vi "CAP Forward Masking.vi"(11 "State":T7={"Experimenter"="XYZ", "Number"=999, "Right"="Right", "Left"="Left", "Data Folder"=path "C:/Data/XYZ DATA/XYZ999", "State File"=path "C:/Data/XYZ DATA/XYZ999/Experiment State.txt", "Version Info"="CFTS VIs: V1.2 (Rev. 132)\nExperiment VIs: 132\nLabVIEW.exe V10.0 (2010)\nDAQmx V9.1", "End Exposure Time"=-1.0, "Exposure Duration"="", "Run #"={"CAP"=0, "ABR"=0, "DP"=0, "VsEP"=0, "MeasSeq"=0, "SubSeq"=0, "SFOAE"=0}}) -> (3 "State Out":T7={"Experimenter"="XYZ", "Number"=999, "Right"="Right", "Left"="Left", "Data Folder"=path "C:/Data/XYZ DATA/XYZ999", "State File"=path "C:/Data/XYZ DATA/XYZ999/Experiment State.txt", "Version Info"="CFTS VIs: V1.2 (Rev. 132)\nExperiment VIs: 132\nLabVIEW.exe V10.0 (2010)\nDAQmx V9.1", "End Exposure Time"=-1.0, "Exposure Duration"="", "Run #"={"CAP"=0, "ABR"=0, "DP"=0, "VsEP"=0, "MeasSeq"=0, "SubSeq"=0, "SFOAE"=0}})   [LabVIEW 2020]
uses:
  CFTS Main Panel SubVIs/CFTS-Experiment State.ctl
  epl-vi-lib/Utility VIs/Type Defs/Left-Right ring.ctl
  Typedefs/CAPFM-Control References.ctl
  Typedefs/CAPFM-All Params.ctl
  Typedefs/CAPFM-Probe Params.ctl
  Typedefs/CAPFM-Masker Params.ctl
  Typedefs/CAPFM-Seq Params.ctl
  Typedefs/CAPFM-Timing Params.ctl
  Typedefs/CAPFM-Response Params.ctl
panel:
  out "Pause Msg":string
  in  "Pause":bool
  out "Attempted":i32
  in  "OverRide":bool
  in  "Threshold (uV)":dbl=15.0
  out "Reject":bool
  out "Decr":cluster{"Interval":dbl[], "Decrement":dbl[]}(graph)
  out "Refs":T1
  out "Mags":cluster{dbl[], dbl[]}[](graph)
  out "CAP":cluster{i32, "dx":dbl, "Array":dbl[][]}(graph)
  in  "Notes":string
  in  "Response":T2={"Gain"=10000.0, "Fs (Hz)"=0.0, "Save traces?"=FALSE, "Window (ms)"=8.0, "Filter?"=FALSE}
  out "Acquired":i32
  out "Interval (ms)":dbl
  in  "Timing":T3={"Rep rate (Hz)"=0.0, "TRecover (ms)"=200.0, "Method"=0} {"Method" items=["Recovery (ms)", "Rep rate (/s)"]}
  in  "Probe":T4={"Freq (kHz)"=10.0, "dB SPL"=50.0, "AltPol"=TRUE, "Dur (ms)"=5.0}
  in  "Sequence":cluster{"Intervals (ms)":string, "NAvgs":i32}={"Intervals (ms)"="2;4;8;16;32;64;128;256;512", "NAvgs"=10}
  in  "Ear":T5
  in  "Masker":T6={"dB SPL"=50.0, "Dur (ms)"=100.0, "InvFilt"=FALSE}
  out "User":string="XYZ"
  out "Run #":u16
  out "ID #":u16=999
  out "running":bool
  in  "Exit":bool
  in  "Go":bool
  out "exit signal":bool
  out "Abort":bool
  in  "Stop":bool
  # "Probe"
  # "Masker"
  # "Intervals"
  # "Response"
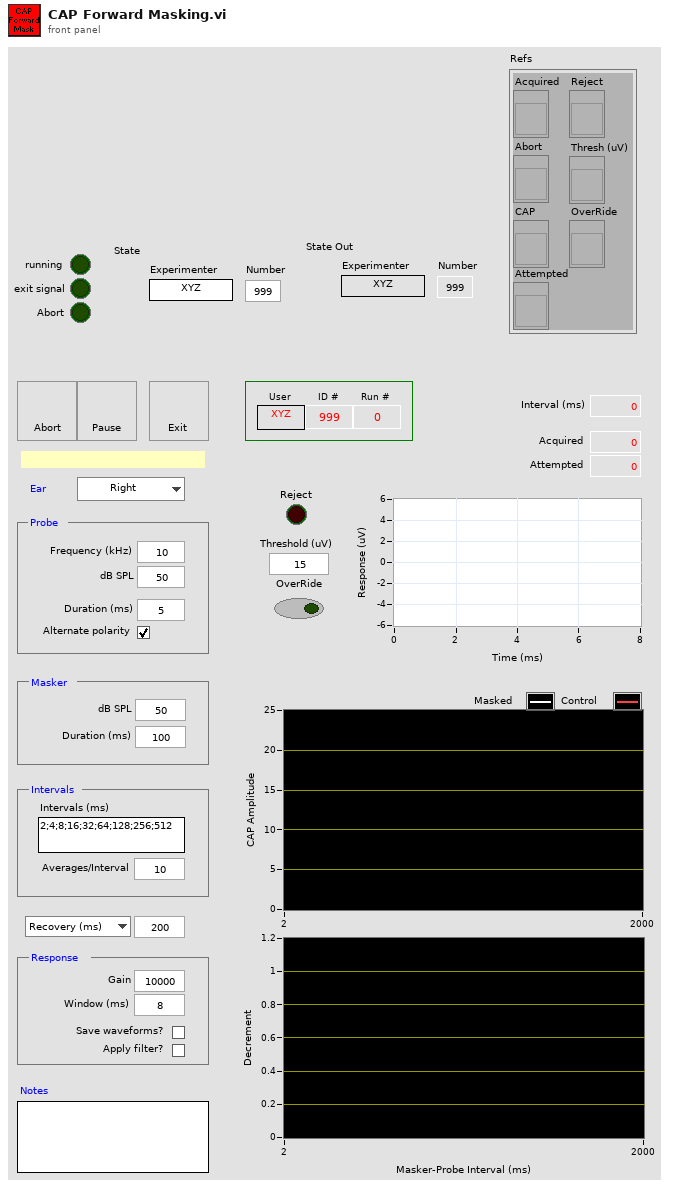
[diagram p1: front panel]
types:
  T1 = typedef "CAPFM-Control References.ctl" = cluster{"Acquired":refnum<vi>, "Abort":refnum<vi>, "CAP":refnum<vi>, "Reject":refnum<vi>, "Thresh (uV)":refnum<vi>, "OverRide":refnum<vi>, "Attempted":refnum<vi>}
  T2 = cluster{"Gain":dbl, "Fs (Hz)":dbl, "Save traces?":bool, "Window (ms)":dbl, "Filter?":bool}
  T3 = cluster{"Rep rate (Hz)":dbl, "TRecover (ms)":dbl, "Method":u16}
  T4 = cluster{"Freq (kHz)":dbl, "dB SPL":dbl, "AltPol":bool, "Dur (ms)":dbl}
  T5 = typedef "Left-Right ring.ctl" = enum16{"Right", "Left"}
  T6 = cluster{"dB SPL":dbl, "Dur (ms)":dbl, "InvFilt":bool}
  T7 = typedef "CFTS-Experiment State.ctl" = cluster{"Experimenter":string, "Number":u32, "Right":string, "Left":string, "Data Folder":path, "State File":path, "Version Info":string, "End Exposure Time":dbl, "Exposure Duration":string, "Run #":cluster{"CAP":i16, "ABR":i16, "DP":i16, "VsEP":i16, "MeasSeq":i16, "SubSeq":i16, "SFOAE":i16}}
  T8 = typedef "CAPFM-All Params.ctl" = cluster{"Ear":T5, "Probe":T9, "Masker":T10, "Sequence":T11, "Fs (Hz)":dbl, "Timing":T12, "Response":T13}
  T9 = typedef "CAPFM-Probe Params.ctl" = cluster{"Freq (kHz)":dbl, "dB SPL":dbl, "AltPol":bool, "Dur (ms)":dbl}
  T10 = typedef "CAPFM-Masker Params.ctl" = cluster{"dB SPL":dbl, "Dur (ms)":dbl, "InvFilt":bool}
  T11 = typedef "CAPFM-Seq Params.ctl" = cluster{"List (ms)":string, "NAvgs":i32}
  T12 = typedef "CAPFM-Timing Params.ctl" = cluster{"Rep rate (Hz)":dbl, "TRecover (ms)":dbl, "Method":enum16{"Fixed recovery", "Fixed rep rate"}}
  T13 = typedef "CAPFM-Response Params.ctl" = cluster{"Gain":dbl, "Fs (Hz)":dbl, "Save traces?":bool, "Window (ms)":dbl, "Filter?":bool}
  T14 = typedef "CAPFM-Runtime Data.ctl" = cluster{"Offset":i32, "AI Npts":i32, "Gain":dbl, "WinPts":i32, "NAvg":i32, "dt (ms)":dbl, "FiltCoef":dbl[]}
  T15 = typedef "Stimulus Channel (Full).xctl/Full Stimulus Channel Data.ctl" = cluster{"Waveform":T16, "Filter":T33, "Burst":T35, "Level":T36, "Name":string, "Advanced":T38, "SAM":T39}
  T16 = typedef "Waveform XCtl.xctl/Waveform Data.ctl" = cluster{"Type":T17, "Tone":T18, "Pulse Train":T19, "Noise":T22, "File":T23, "FMSweep":T24, "Chirp Train":T25, "Complex Tone":cluster{"Params":T27, "Data":T29}, "Moving Ripple":T30}
  T17 = typedef "Waveform Enum.ctl" = enum16{"OFF", "Tone", "Noise", "Pulse Train", "File", "FM Sweep", "Chirp Train", "Complex Tone", "FM Tone", "Moving Ripple"}
  T18 = typedef "Tone Params.ctl" = cluster{"Frequency (kHz)":dbl, "Last Freq":dbl, "Last Phase":dbl}
  T19 = typedef "Pulse Train Params.ctl" = cluster{"Pulse width (us)":dbl, "Pulse rate (Hz)":dbl, "Gap (ms)":dbl, "Polarity":T20, "PT State":T21, "Asynch":bool}
  T20 = typedef "Pulse Polarity.ctl" = enum16{"POS", "NEG", "POS-NEG", "NEG-POS"}
  T21 = typedef "PT-Continuous State.ctl" = cluster{"Template":dbl[], "Nperiod":i32, "Index":i32, "Pulse Rate (Hz)":dbl, "Phase (cycles)":dbl, "Noff":i32}
  T22 = typedef "Noise Params.ctl" = cluster{"InvFilt":bool, "Noise":dbl[], "CurPt":i32, "Aweight":bool, "Seed":i32, "afile":path}
  T23 = typedef "StimFile-Params.ctl" = cluster{"Filename":path, "Signal":dbl[], "Channel":i32, "stream":bool, "offset":i32, "nreps":i32, "loops":i32, "Randomize":bool, "order":i32[], "Seed":i32, "Tokens":i32}
  T24 = typedef "FM Sweep Params.ctl" = cluster{"Rate (oct/s)":dbl, "Fmin (Hz)":dbl, "Fmax (Hz)":dbl, "Ramp (ms)":dbl, "Linear":bool}
  T25 = typedef "Chirp Train.ctl" = cluster{"Params":T26, "Data":cluster{"WF":dbl[]}}
  T26 = typedef "Chirp Train Params.ctl" = cluster{"Fmin (kHz)":dbl, "Fmax (kHz)":dbl, "Compensate":bool, "Duration (ms)":dbl}
  T27 = typedef "CT-Params.ctl" = cluster{"F0 (Hz)":dbl, "Band":cluster{"Flow (Hz)":dbl, "Fhigh (Hz)":dbl}, "Phase":T28, "Min F0 (Hz)":dbl, "Max F0 (Hz)":dbl, "ContinRandPhase":bool, "Max peak factor":dbl, "Max mod depth":dbl, "MinHarmNum":i32, "MaxHarmNum":i32, "Level Mode":enum16{"per component", "overall rms"}, "% jitter":dbl}
  T28 = typedef "CT-Phase Enum.ctl" = enum16{"Cosine", "Random", "Alternating"}
  T29 = typedef "CT-Runtime Data.ctl" = cluster{"Ncomp":i32, "MinHarm":i32, "Phase":dbl[], "Amplitude":dbl[], "Npts/frame":i32, "Last F0":dbl, "Fmin":dbl, "Fmax":dbl, "Lslope":dbl, "randphase":bool, "overall rms":bool, "fmult":dbl[], "jittered":bool}
  T30 = typedef "Moving Ripple.ctl" = cluster{"Params":T31, "Data":T32}
  T31 = typedef "Moving Ripple.Params.ctl" = cluster{"Fmin":dbl, "Fmax":dbl, "Density":dbl, "Velocity":dbl, "Depth":dbl, "Phase":dbl, "Comp/oct":i32}
  T32 = typedef "Moving Ripple.Data.ctl" = cluster{"Freq":dbl[], "A":dbl[], "phase":dbl[], "Phase":dbl}
  T33 = typedef "Advanced Filter XCtl.xctl/Filter Data.ctl" = cluster{"Type":enum16{"Lowpass", "Highpass", "Bandpass", "Bandstop", "OFF"}, "CF (kHz)":dbl, "BW (kHz)":dbl, "Cascade":bool, "Quadrature":bool, "Scale Factor":dbl, "Stages":cluster{"IIR Filter":cluster{"filter structure":enum32{"IIR 2nd Order", "IIR 4th Order"}, "Reverse Coefficients":dbl[], "Forward Coefficients":dbl[]}, "State":dbl[]}[], "Class":enum16{"Elliptic", "Butterworth"}, "Order":i32, "BWUnits":T34}
  T34 = typedef "Filter-Bandwidth Units.ctl" = enum16{"Linear", "Octaves", "Min-Max"}
  T35 = typedef "Burst Control.xctl/Burst Data.ctl" = cluster{"Active":bool, "Delay (ms)":dbl, "Duration (ms)":dbl, "Ramp (ms)":dbl, "Rate (Hz)":dbl, "Trepeat (ms)":dbl, "Repeat":bool}
  T36 = typedef "Level XCtl.xctl/Level Data.ctl" = cluster{"Level":dbl, "Units":T37, "Max":dbl, "Multiplier":dbl, "Cal File":path, "Cal":cluster{"Freq (Hz)":dbl[], "Mag (dB SPL)":dbl[], "Phase (deg)":dbl[]}}
  T37 = typedef "Level Units.ctl" = enum16{"dB atten", "dB SPL", "dB re 1 Vrms", "dB V/Hz½", "mW", "dB HL", "Volts", "dB mW"}
  T38 = typedef "Advanced Stimulus Options.xctl/Advanced Stimulus Options.ctl" = cluster{"Rep Mask":string, "AltPol":bool, "Var":string, "Expr":string, "Persist":bool}
  T39 = typedef "SAM Params.ctl" = cluster{"Active":bool, "Frequency (Hz)":dbl, "Depth":dbl, "Init Phase (cycles)":dbl, "phase (degrees)":dbl, "Asynch":bool}
  T40 = typedef "CAPFM-Analysis State.ctl" = cluster{"CAPs":dbl[][], "Interval":dbl[], "Control":dbl[], "Masked":dbl[], "Decrement":dbl[], "Order":i32[]}
  T41 = cluster{"Acquired":refnum<vi>, "Abort":refnum<vi>, "CAP":refnum<vi>, "Reject":refnum<vi>, "Threshold (uV)":refnum<vi>, "OverRide":refnum<vi>, "Attempted":refnum<vi>}
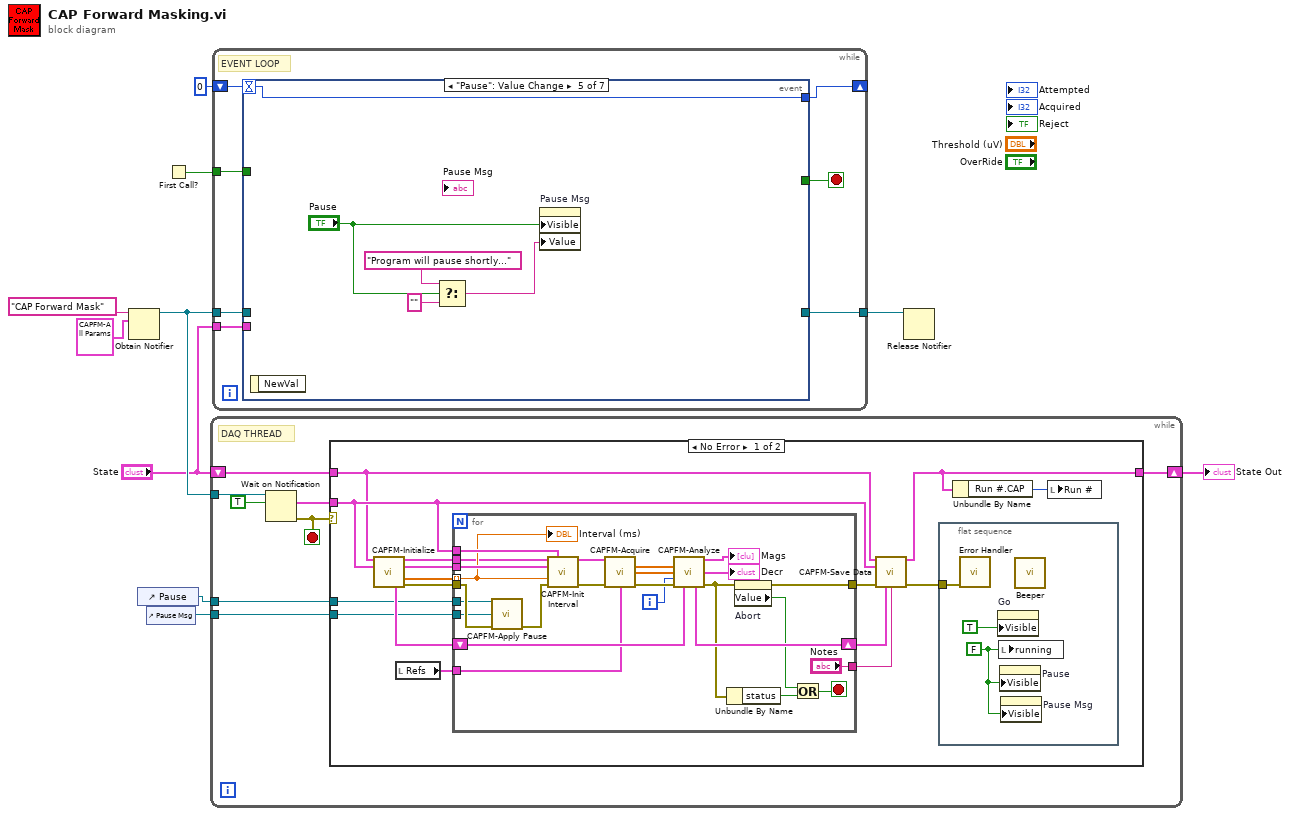
[diagram p0: block diagram]
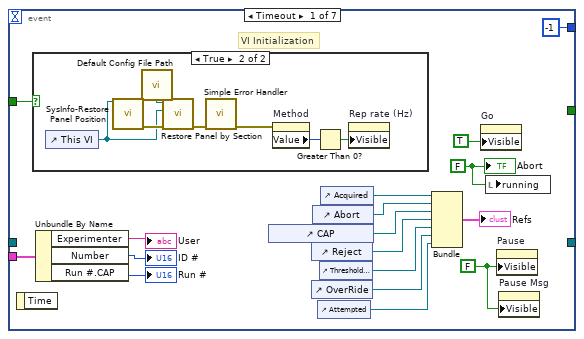
[diagram p3: hidden frame]
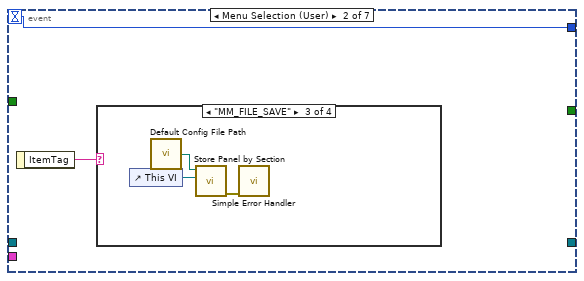
[diagram p5: hidden frame]
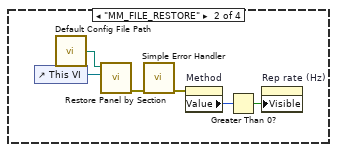
[diagram p7: hidden frame]
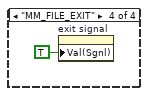
[diagram p8: hidden frame]
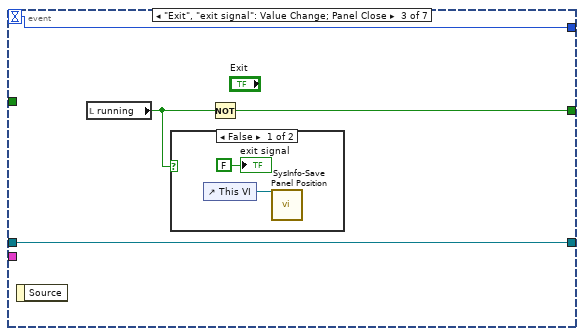
[diagram p9: hidden frame]
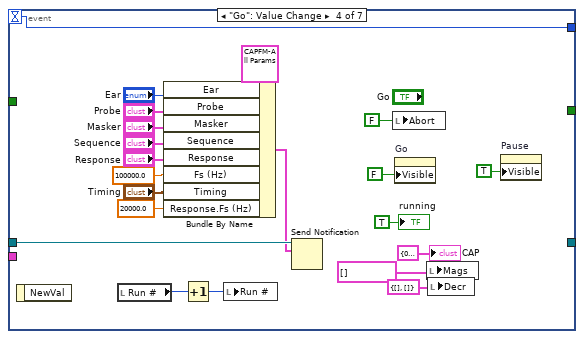
[diagram p11: hidden frame]
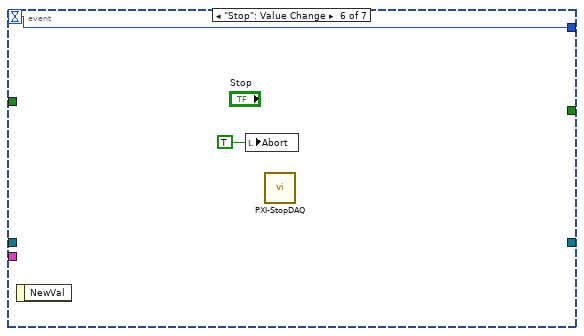
[diagram p12: hidden frame]
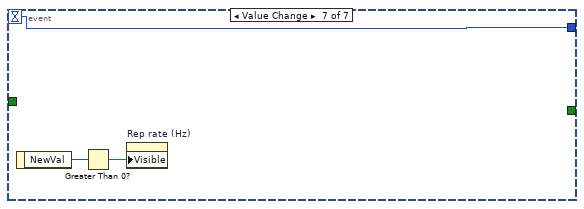
[diagram p13: hidden frame]
diagram:
  n1 = Obtain Notifier(name (unnamed)="CAP Forward Mask", notification data type=T8 {"Ear"=enum."Right", "Probe"={"Freq (kHz)"=0.0, "dB SPL"=0.0, "AltPol"=FALSE, "Dur (ms)"=0.0}, "Masker"={"dB SPL"=0.0, "Dur (ms)"=0.0, "InvFilt"=FALSE}, "Sequence"={"List (ms)"="", "NAvgs"=0}, "Fs (Hz)"=0.0, "Timing"={"Rep rate (Hz)"=0.0, "TRecover (ms)"=0.0, "Method"=enum."Fixed recovery"}, "Response"={"Gain"=0.0, "Fs (Hz)"=0.0, "Save traces?"=FALSE, "Window (ms)"=0.0, "Filter?"=FALSE}} ("CAPFM Params")) -> (notifier out=w6:refnum<notifier>)  [unwired: 2 in, 2 out]
  n2 = control-ref of="Pause"() -> (w2:refnum<vi>)
  n3 = control-ref of="Pause Msg"() -> (w1:refnum<vi>)
  n4 = First Call?() -> (First Call?: T/F=w7:bool)
  n5 = while {
    tunnel: w6 -> [w17]
    shift-right: [w13] -> w3
    shift-left: "State" -> [w14]
    tunnel: w2 -> [w12]
    tunnel: w1 -> [w11]
    stop <- w15 stop-if-true
    # "DAQ THREAD"
    n6 = Wait on Notification(notifier=w17, ignore previous (F)=TRUE) -> (notification=w16:T8, error out=w15:errorcluster)  [unwired: 2 in, 2 out]
    n7 = case shown="No Error" w15 {
      tunnel: w16 -> [w27 _]
      tunnel: w14 -> [w26 w63]
      tunnel: [w25 w63] -> w13
      tunnel: w12 -> [w20 _]
      tunnel: w11 -> [w19 _]
      frame No Error {
        n8 = call "CAPFM-Initialize.vi"("Expt State"=w26, "CAPFM Params"=w27) -> ("Runtime"=w21:T14, "StimChans"=w31:T15[], "Intervals (ms)"=w34:dbl[], "Analysis"=w33:T40, "error out"=w32:errorcluster)  [unwired: 9 in]
        n9 = local read "Refs"() -> (w22:T1)
        n10 = for {
          tunnel: w34 -> [w40] mode=indexing
          shift-right: [w55] -> w29
          shift-left: w33 -> [w56]
          tunnel: w32 -> [w37]
          tunnel: w31 -> [w59]
          tunnel: w27 -> [w41]
          tunnel: [w43] -> w30
          tunnel: ["Notes"] -> w28
          tunnel: w22 -> [w50]
          tunnel: w21 -> [w39]
          tunnel: w20 -> [w36]
          tunnel: w19 -> [w35]
          i -> [w49]
          stop <- w46 stop-if-true
          n11 = call "CAPFM-Apply Pause.vi"("Pause Ref"=w36, "Pause Msg Ref"=w35, "error in (no error)"=w37) -> ("error out"=w38:errorcluster)  [unwired: 12 in]
          n12 = call "CAPFM-Init Interval.vi"("Runtime In"=w39, "CAPFM Params"=w41, "StimChans"=w59, "Interval (ms)"=w40, "error in (no error)"=w38) -> ("Runtime Out"=w54:T14, "error out"=w58:errorcluster)  [unwired: 9 in]
          n13 = call "CAPFM-Acquire.vi"("Runtime"=w54, "error in (no error)"=w58, "Refs"=w50) -> ("Control"=w53:dbl[], "Masked"=w52:dbl[], "error out"=w57:errorcluster)  [unwired: 10 in]
          n14 = call "CAPFM-Analyze.vi"("Control"=w53, "Masked"=w52, "Index"=w49, "error in (no error)"=w57, "Analysis"=w56) -> ("Mags"=→"Mags":cluster{"Interval":dbl[], "Control":dbl[]}[], "Decrement"=→"Decr":cluster{"Interval":dbl[], "Decrement":dbl[]}, "Analysis Out"=w55:T40, "error out"=w47:errorcluster)  [unwired: 7 in]
          n15 = Unbundle By Name(w47) -> ("status"=w45:bool)
          n16 = property on="Abort" class="Bool (strict)"(error in=w47) -> (error out=w43:errorcluster, "Value"=w42:bool)  [unwired: 1 in, 1 out]
          n17 = Or(x=w42, y=w45) -> (x .or. y?=w46:bool)
          "Interval (ms)" <- w40
        }
        n18 = call "CAPFM-Save Data.vi"("Expt State"=w26, "CAPFM Params"=w27, "error in"=w30, "Analysis"=w29, "Notes"=w28) -> ("Expt State Out"=w25:T7, "error out"=w23:errorcluster)  [unwired: 9 in]
        n19 = flat-sequence {
          tunnel: w23 -> [w61]
          frame #0 {
            w60 = FALSE ("running")
            n20 = call "Error Handler.vi"("error in (no error)"=w61) -> ()  [unwired: 13 in, 2 out]
            n21 = property on="Go" class="Bool"("Visible"=TRUE) -> ()  [unwired: 2 in, 2 out]
            n22 = local write "running"(w60) -> ()
            n23 = property on="Pause" class="Bool (strict)"("Visible"=w60) -> ()  [unwired: 2 in, 2 out]
            n24 = property on="Pause Msg" class="Str"("Visible"=w60) -> ()  [unwired: 2 in, 2 out]
            n25 = call "Beeper.vi"() -> ()  [unwired: 5 in, 1 out]
          }
        }
        n26 = Unbundle By Name(w25) -> ("Run #.CAP"=w24:i16)
        n27 = local write "Run #"(w24) -> ()
      }
      frame Error {
      }
    }
  }
  "State Out" <- w3
  n28 = while {
    tunnel: w6 -> [w70]
    tunnel: [w68] -> w10
    shift-right: [w66] -> _
    shift-left: 0 -> [w67]
    tunnel: w7 -> [w65]
    tunnel: "State" -> [w64]
    stop <- w69 stop-if-true
    # "EVENT LOOP"
    n29 = event shown="[4] \"Pause\": Value Change" {
      selector: _ -> [_ _ _ _ _ _ _]
      dyn-events: _ -> [_ _ _ _ _ _ _]
      timeout: w67 -> [_ w95 w109 w131 w138 w139 w143]
      tunnel: w70 -> [_ _ w110 w133 _ _ _]
      tunnel: [_ _ w107 _ _ _ _] -> w69
      tunnel: [_ _ w110 _ _ _ _] -> w68
      tunnel: [-1 w95 w109 w131 w138 w139 w143] -> w66
      tunnel: w65 -> [w84 _ _ _ _ _ _]
      tunnel: w64 -> [w83 _ _ _ _ _ _]
      event Timeout {
        w71 = FALSE ("Visible")
        w85 = FALSE ("Abort")
        # "VI Initialization"
        n30 = event-data() -> ()  [unwired: 1 in, 1 out]
        n31 = case shown="True" w84 {
          frame False {
          }
          frame True {
            n32 = control-ref of="This VI"() -> (w88:refnum<vi>)
            n33 = call "SysInfo-Restore Panel Position.vi"("VI Refnum"=w88) -> ("error out"=w92:errorcluster)  [unwired: 12 in, 2 out]
            n34 = call "Default Config File Path.vi"() -> ("Default config file name"=w93:path)
            n35 = call "Restore Panel by Section.vi"("error in (no error)"=w92, "VI reference"=w88, "Path (dialog)"=w93) -> ("Error Out"=w94:errorcluster)  [unwired: 8 in]
            n36 = call <vilib>:"Simple Error Handler.vi"("error in (no error)"=w94) -> ("error out"=w91:errorcluster)  [unwired: 4 in, 4 out]
            n37 = property on="Method" class="Ring (strict)"(error in=w91) -> ("Value"=w89:u16)  [unwired: 1 in, 2 out]
            n38 = Greater Than 0?(x=w89) -> (x > 0?=w90:bool)
            n39 = property on="Rep rate (Hz)" class="DigNum (strict)"("Visible"=w90) -> ()  [unwired: 2 in, 2 out]
          }
        }
        n40 = Unbundle By Name(w83) -> ("Experimenter"=→"User":string, "Number"=→"ID #":u32, "Run #.CAP"=→"Run #":i16)
        n41 = control-ref of="CAP"() -> (w77:refnum<vi>)
        n42 = control-ref of="Reject"() -> (w74:refnum<vi>)
        n43 = control-ref of="OverRide"() -> (w76:refnum<vi>)
        n44 = control-ref of="Abort"() -> (w78:refnum<vi>)
        n45 = control-ref of="Attempted"() -> (w73:refnum<vi>)
        n46 = control-ref of="Threshold (uV)"() -> (w75:refnum<vi>)
        n47 = control-ref of="Acquired"() -> (w79:refnum<vi>)
        n48 = Bundle("Acquired"=w79, "Abort"=w78, "CAP"=w77, "Reject"=w74, "Threshold (uV)"=w75, "OverRide"=w76, "Attempted"=w73) -> (→"Refs":T41)  [unwired: 1 in]
        n49 = property on="Go" class="Bool"("Visible"=TRUE) -> ()  [unwired: 2 in, 2 out]
        n50 = local write "running"(w85) -> ()
        n51 = property on="Pause" class="Bool (strict)"("Visible"=w71) -> ()  [unwired: 2 in, 2 out]
        n52 = property on="Pause Msg" class="Str"("Visible"=w71) -> ()  [unwired: 2 in, 2 out]
        "Abort" <- w85
      }
      event Menu Selection (User) {
        n53 = event-data() -> ("ItemTag"=w96:string)  [unwired: 1 in]
        n54 = case shown="\"MM_FILE_SAVE\"" w96 {
          frame "False", Default {
          }
          frame "MM_FILE_RESTORE" {
            n55 = control-ref of="This VI"() -> (w101:refnum<vi>)
            n56 = call "Default Config File Path.vi"() -> ("Default config file name"=w100:path)
            n57 = call "Restore Panel by Section.vi"("VI reference"=w101, "Path (dialog)"=w100) -> ("Error Out"=w102:errorcluster)  [unwired: 9 in]
            n58 = call <vilib>:"Simple Error Handler.vi"("error in (no error)"=w102) -> ("error out"=w97:errorcluster)  [unwired: 4 in, 4 out]
            n59 = property on="Method" class="Ring (strict)"(error in=w97) -> ("Value"=w99:u16)  [unwired: 1 in, 2 out]
            n60 = Greater Than 0?(x=w99) -> (x > 0?=w98:bool)
            n61 = property on="Rep rate (Hz)" class="DigNum (strict)"("Visible"=w98) -> ()  [unwired: 2 in, 2 out]
          }
          frame "MM_FILE_SAVE" {
            n62 = control-ref of="This VI"() -> (w104:refnum<vi>)
            n63 = call "Default Config File Path.vi"() -> ("Default config file name"=w103:path)
            n64 = call "Store Panel by Section.vi"("VI reference"=w104, "Path (dialog)"=w103) -> ("Error Out"=w105:errorcluster)  [unwired: 9 in]
            n65 = call <vilib>:"Simple Error Handler.vi"("error in (no error)"=w105) -> ()  [unwired: 4 in, 5 out]
          }
          frame "MM_FILE_EXIT" {
            n66 = property on="exit signal" class="Bool (strict)"("Val(Sgnl)"=TRUE ("Value (Signaling)")) -> ()  [unwired: 2 in, 2 out]
          }
        }
      }
      event "Exit", "exit signal": Value Change; Panel Close {
        n67 = event-data() -> ()  [unwired: 1 in, 1 out]
        n68 = local read "running"() -> (w108:bool)
        n69 = case shown="False" w108 {
          frame False {
            n70 = control-ref of="This VI"() -> (w111:refnum<vi>)
            n71 = call "SysInfo-Save Panel Position.vi"("VI Refnum"=w111) -> ()  [unwired: 14 in, 1 out]
            "exit signal" <- FALSE ("exit signal")
          }
          frame True {
          }
        }
        n72 = Not(x=w108) -> (.not. x?=w107:bool)
      }
      event "Go": Value Change {
        n73 = event-data() -> ()  [unwired: 1 in, 1 out]
        n74 = local read "Run #"() -> (w119:u16)
        n75 = Bundle By Name(cluster=T8 {"Ear"=enum."Right", "Probe"={"Freq (kHz)"=0.0, "dB SPL"=0.0, "AltPol"=FALSE, "Dur (ms)"=0.0}, "Masker"={"dB SPL"=0.0, "Dur (ms)"=0.0, "InvFilt"=FALSE}, "Sequence"={"List (ms)"="", "NAvgs"=0}, "Fs (Hz)"=0.0, "Timing"={"Rep rate (Hz)"=0.0, "TRecover (ms)"=0.0, "Method"=enum."Fixed recovery"}, "Response"={"Gain"=0.0, "Fs (Hz)"=0.0, "Save traces?"=FALSE, "Window (ms)"=0.0, "Filter?"=FALSE}} ("CAPFM Params"), "Ear"="Ear", "Probe"="Probe", "Masker"="Masker", "Sequence"="Sequence", "Response"="Response", "Fs (Hz)"=100000.0, "Timing"="Timing", "Response.Fs (Hz)"=20000.0) -> (w129:T8)
        n76 = Increment(x=w119) -> (x+1=w118:u16)
        n77 = local write "Run #"(w118) -> ()
        n78 = Send Notification(notification=w129, notifier=w133) -> ()  [unwired: 1 in, 2 out]
        n79 = local write "Abort"(FALSE ("Abort")) -> ()
        n80 = property on="Go" class="Bool"("Visible"=FALSE) -> ()  [unwired: 2 in, 2 out]
        n81 = local write "Mags"(cluster{dbl[], dbl[]}[] [] ("Mags")) -> ()
        n82 = local write "Decr"(cluster{"Interval":dbl[], "Decrement":dbl[]} {"Interval"=[], "Decrement"=[]} ("Decr")) -> ()
        n83 = property on="Pause" class="Bool (strict)"("Visible"=TRUE) -> ()  [unwired: 2 in, 2 out]
        "running" <- TRUE ("running")
        "CAP" <- cluster{i32, "dx":dbl, "Array":dbl[][]} {0, "dx"=0.05, "Array"=[]} ("CAP")
      }
      event "Pause": Value Change {
        n84 = event-data() -> ()  [unwired: 1 in, 1 out]
        n85 = Select(t="Program will pause shortly...", s="Pause", f="") -> (s? t:f=w134:string)
        n86 = property on="Pause Msg" class="Str"("Visible"="Pause", "Value"=w134) -> ()  [unwired: 2 in, 2 out]
      }
      event "Stop": Value Change {
        n87 = event-data() -> ()  [unwired: 1 in, 1 out]
        n88 = local write "Abort"(TRUE ("Abort")) -> ()
        n89 = call "PXI-StopDAQ.vi"() -> ()  [unwired: 7 in, 1 out]
      }
      event "Timing.Method": Value Change {
        n90 = event-data() -> ("NewVal"=w142:u16)  [unwired: 1 in]
        n91 = Greater Than 0?(x=w142) -> (x > 0?=w141:bool)
        n92 = property on="Rep rate (Hz)" class="DigNum (strict)"("Visible"=w141) -> ()  [unwired: 2 in, 2 out]
      }
    }
  }
  n93 = Release Notifier(notifier=w10) -> ()  [unwired: 2 in, 3 out]
